vi "Get Library Classes from This Project.vi"(8 "error in (no error)":errorcluster, 10 "Target Name (My Computer)":string="My Computer", 11 "Library Name":string) -> (0 "error out":errorcluster)   [LabVIEW 2017, in "Build Automation.lvlib"]
uses:
  Build Automation.lvlib
panel:
  out "class refs":refnum<vi>[](array[refnum])
  out "class names":string[](array[string])
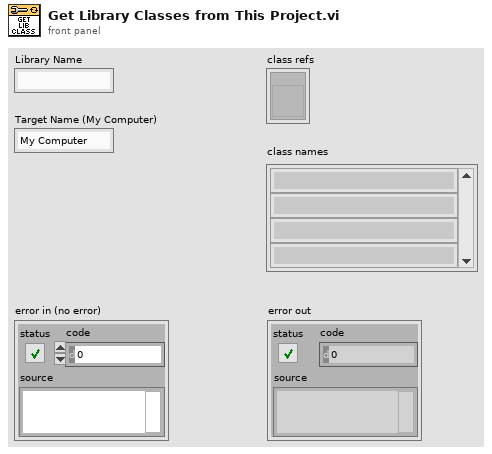
[diagram p1: front panel]
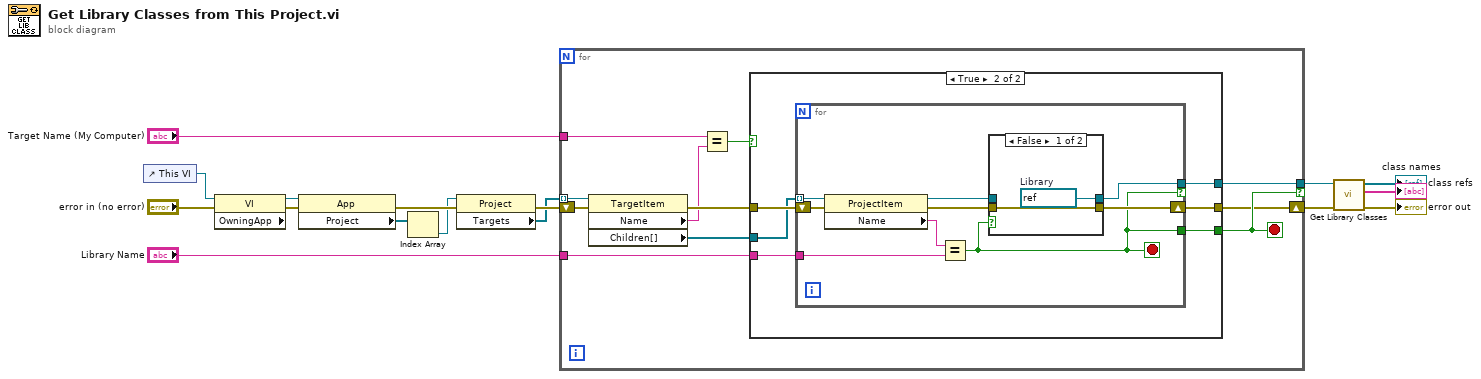
[diagram p0: block diagram]
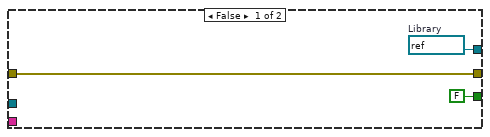
[diagram p2: hidden frame]
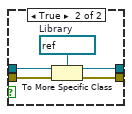
[diagram p3: hidden frame]
diagram:
  n1 = control-ref of="This VI"() -> (w16:refnum<vi>)
  n2 = property class="VI"(reference=w16, error in="error in (no error)") -> (error out=w9:errorcluster, "OwningApp"=w15:refnum<vi>)  [unwired: 1 out]
  n3 = property class="App"(reference=w15, error in=w9) -> (error out=w11:errorcluster, "Project"=w14:refnum<vi>[])  [unwired: 1 out]
  n4 = Index Array(array=w14) -> (element=w10:refnum<vi>)  [unwired: 1 in]
  n5 = property class="Project"(reference=w10, error in=w11) -> (error out=w8:errorcluster, "Targets"=w7:refnum<vi>[])  [unwired: 1 out]
  n6 = for {
    tunnel: w7 -> [w27] mode=indexing
    tunnel: "Library Name" -> [w26]
    tunnel: [w25] -> w5 if=w24
    shift-right: [w23] -> w4
    shift-left: w8 -> [w22]
    tunnel: "Target Name (My Computer)" -> [w18]
    stop <- w24 stop-if-true
    n7 = property class="TargetItem"(reference=w27, error in=w22) -> (error out=w21:errorcluster, "Name"=w19:string, "Children[]"=w20:refnum<vi>[])  [unwired: 1 out]
    n8 = Equal?(x=w18, y=w19) -> (x = y?=w17:bool)
    n9 = case shown="True" w17 {
      tunnel: w26 -> [_ w36]
      tunnel: [w30 w35] -> w25
      tunnel: [FALSE w34] -> w24
      tunnel: [w28 w33] -> w23
      tunnel: w21 -> [w28 w32]
      tunnel: w20 -> [_ w31]
      frame False {
        w30 = refnum<vi> refnum  # Library
      }
      frame True {
        n10 = for {
          tunnel: w31 -> [w45] mode=indexing
          tunnel: w36 -> [w43]
          tunnel: [w39] -> w35 if=w37
          shift-right: [w41] -> w33
          shift-left: w32 -> [w38]
          tunnel: [w37] -> w34
          stop <- w37 stop-if-true
          n11 = property class="ProjectItem"(reference=w45, error in=w38) -> (reference out=w40:refnum<vi>, error out=w42:errorcluster, "Name"=w44:string)
          n12 = Equal?(x=w44, y=w43) -> (x = y?=w37:bool)
          n13 = case shown="False" w37 {
            tunnel: w42 -> [w47 w52]
            tunnel: [w47 w51] -> w41
            tunnel: w40 -> [_ w50]
            tunnel: [w46 w49] -> w39
            frame False {
              w46 = refnum<vi> refnum  # Library
            }
            frame True {
              w48 = refnum<vi> refnum  # Library
              n14 = To More Specific Class(target class=w48, reference=w50, error in=w52) -> (specific class reference=w49:refnum<vi>, error out=w51:errorcluster)
            }
          }
        }
      }
    }
  }
  n15 = call "Get Library Classes.vi"("error in (no error)"=w4, "library ref"=w5) -> ("error out"=→"error out":errorcluster, "class names"=→"class names":string[], "class refs"=→"class refs":refnum<vi>[])  [unwired: 7 in]
